vi "Pre-Build CHM Build.vi"(8 "error in (no error)":errorcluster, 11 "Main Destination Path":path) -> (0 "error out":errorcluster)   [LabVIEW 2019]
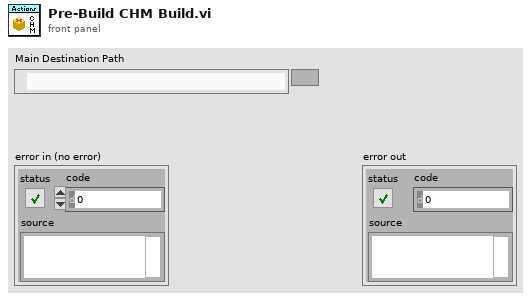
[diagram p1: front panel]
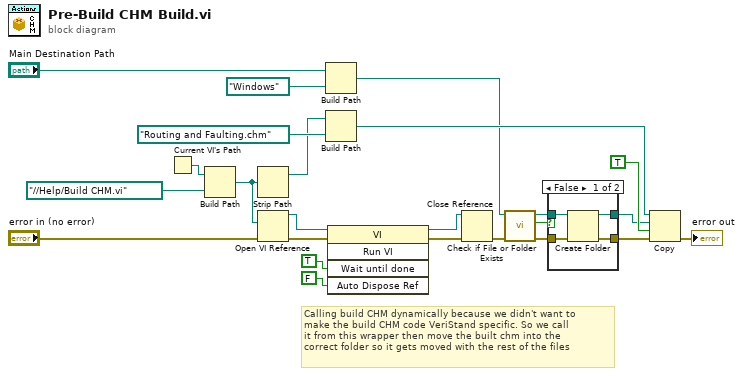
[diagram p0: block diagram]
diagram:
  # "Calling build CHM dynamically because we didn't want to \nmake the build CHM code VeriStand specific. So we call\nit from this wrapper then move the built chm into the\ncorrect folder so it gets moved with the rest of the files"
  n1 = Current VI's Path() -> (path=w2:path)
  n2 = Build Path(base path=w2, name or relative path=path "../../Help/Build CHM.vi") -> (appended path=w10:path)
  n3 = Strip Path(path=w10) -> (stripped path=w23:path)  [unwired: 1 out]
  n4 = Open VI Reference(vi path=w10, error in (no error)="error in (no error)") -> (vi reference=w4:refnum<vi>, error out=w5:errorcluster)  [unwired: 4 in]
  n5 = Build Path(base path="Main Destination Path", name or relative path=path "Windows") -> (appended path=w13:path)
  n6 = Build Path(base path=w23, name or relative path=path "Routing and Faulting.chm" ("stripped path")) -> (appended path=w21:path)
  n7 = invoke class="VI" method="Run VI"(reference=w4, error in=w5, "Wait until done"=TRUE ("Wait Until Done"), "Auto Dispose Ref"=FALSE ("Auto Dispose Reference")) -> (reference out=w8:refnum<vi>, error out=w9:errorcluster)  [unwired: 1 in, 3 out]
  n8 = Close Reference(reference=w8, error in (no error)=w9) -> (error out=w14:errorcluster)
  n9 = call <vilib>:"Check if File or Folder Exists.vi"("error in (no error)"=w14, "path"=w13) -> ("error out"=w17:errorcluster, "file or folder exists?"=w15:bool, "dup path"=w16:path)  [unwired: 7 in]
  n10 = case shown="False" w15 {
    tunnel: w16 -> [w27 w30]
    tunnel: w17 -> [w28 w29]
    tunnel: [w26 w30] -> w19
    tunnel: [w25 w29] -> w18
    frame False {
      n11 = Create Folder(path (use dialog)=w27, error in=w28) -> (created path=w26:path, error out=w25:errorcluster)  [unwired: 1 in, 1 out]
    }
    frame True {
    }
  }
  n12 = Copy(8:w18, 9:TRUE ("overwrite (F)"), 10:w19, 11:w21) -> (0:→"error out":errorcluster)  [unwired: 1 in, 2 out]
